vi "str2buffer.vi"(6 "input buffer":u8[](array[numeric]), 7 "string bitmap":u8[](array[numeric]), 8 "y":u8, 9 "x":u8) -> (3 "output buffer":u8[](array[numeric]))   [LabVIEW 2017]
panel:
  out "current byte":bool[](array[boolean])
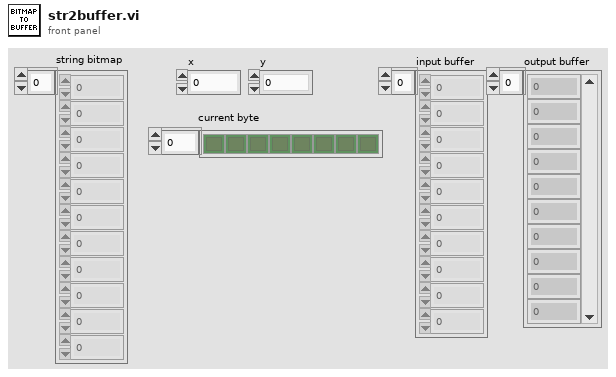
[diagram p1: front panel]
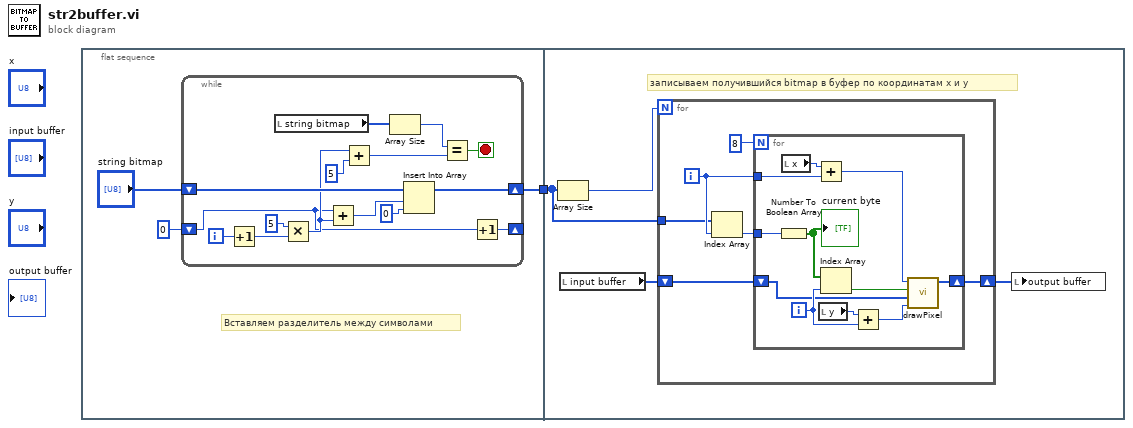
[diagram p0: block diagram]
diagram:
  n1 = flat-sequence {
    tunnel: [w2] -> w1
    tunnel: w1 -> [w20]
    frame #0 {
      # "Вставляем разделитель между символами"
      n2 = while {
        shift-right: [w9] -> w2
        shift-left: "string bitmap" -> [w10]
        shift-right: [w8] -> _
        shift-left: u8 0 -> [w6]
        i -> [w19]
        stop <- w12 stop-if-true
        n3 = Increment(x=w19) -> (x+1=w18:i32)
        n4 = local read "string bitmap"() -> (w14:u8[])
        n5 = Multiply(x=5, y=w18) -> (x*y=w7:i32)
        n6 = Add(x=w6, y=w7) -> (x+y=w5:i32)
        n7 = Add(x=w7, y=5) -> (x+y=w11:i32)
        n8 = Array Size(array=w14) -> (size(s)=w13:i32)
        n9 = Insert Into Array "Insert Into Array"(array=w10, index=w5, new element=u8 0 ("new element/subarray")) -> (w9:u8[])
        n10 = Equal?(x=w13, y=w11) -> (x = y?=w12:bool)
        n11 = Increment(x=w6) -> (x+1=w8:u8)
      }
    }
    frame #1 {
      # "записываем получившийся bitmap в буфер по координатам x и y"
      n12 = Array Size(array=w20) -> (size(s)=w23:i32)
      n13 = local read "input buffer"() -> (w21:u8[])
      n14 = for {
        N: w23 -> [_]
        shift-right: [w27] -> w22
        shift-left: w21 -> [w26]
        tunnel: w20 -> [w25]
        i -> [w28]
        n15 = Index Array "Index Array"(array=w25, index=w28) -> (element=w24:u8)
        n16 = for {
          N: 8 -> [_]
          tunnel: w24 -> [w33]
          tunnel: w28 -> [w35]
          shift-right: [w31] -> w27
          shift-left: w26 -> [w30]
          i -> [w39]
          n17 = Number To Boolean Array(number=w33) -> (Boolean array=w32:bool[])
          "current byte" <- w32
          n18 = local read "x"() -> (w36:u8)
          n19 = Add(x=w36, y=w35) -> (x+y=w34:i32)
          n20 = local read "y"() -> (w38:u8)
          n21 = Index Array "Index Array"(array=w32, index=w39) -> (element=w40:bool)
          n22 = Add(x=w38, y=w39) -> (x+y=w37:i32)
          n23 = call "drawPixel.vi"("y"=w37, "input_buffer"=w30, "color"=w40, "x"=w34) -> ("output_buffer"=w31:u8[])  [unwired: 7 in]
        }
      }
      n24 = local write "output buffer"(w22) -> ()
    }
  }
